vi "Pockels Cal-Init laser power meas.vi"(8 "error in (no error)":errorcluster) -> (0 "error out":errorcluster, 2 "Auto-cancel":bool, 3 "Laser power measrement task":refnum<k21>)   [LabVIEW 2017]
uses:
  Typedefs/HW config states enum.ctl
  <vilib>/DAQmx/create/channels.llb/DAQmx Create Channel (AI-Voltage-Basic).vi
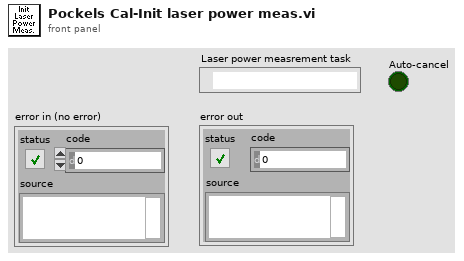
[diagram p1: front panel]
types:
  T1 = typedef "HW config states enum.ctl" = enum16{"Load from file", "Save to file", "Write all", "Read all", "Write XY stage settings", "Write DAQ FPGA settings", "Write Control FPGA settings", "Write Phys Channels", "Clear", "Compare from file"}
  T2 = typedef "Hardware Configuration settings.ctl" = cluster{"Microscope ID":string, "Microscope Type":string, "Revision Number":string, "Advanced Imaging":bool, "Max Allowed Trial Length":dbl, "Initial Scan Resolution":dbl, "Initial Acceptance Angle":dbl, "Dev. PC":bool, "Swap XY on stage":bool, "No of AOD":u8, "MC Supported":bool, "Axial MC":bool, "Computer MAC address":string, "Externalise Triggers":bool, "Trigger HW config":T3, "DAQmx Chan":T4, "XY stage available":bool, "XY Stage":T5, "Z stage available":bool, "Z Stage config cluster":T6, "Encoder available":bool, "Encoder":T7, "VidRec available":bool, "Cam VidRec":T8, "Laser Power Control HW config":T9, "Laser 1 available":bool, "Laser 1 config cluster":T10, "Prechirper 1 available":bool, "Prechirper 1 config cluster":T11, "Control system.FPGA available?":bool, "Control Sys. HW config":T12, "DAQ FPGA HW Config":cluster{"Target":T13, "input card type":T14}}
  T3 = typedef "Triggers HW config.ctl" = cluster{"Available Device List":i32, "Device Address":string}
  T4 = typedef "DAQmx physical channels cluster.ctl" = cluster{"Pockels AO":tag, "Hard shutter AO":tag, "PMT AOs":tag, "Galvo AOs":tag, "Power meter AI":tag}
  T5 = typedef "XY Stage config cluster.ctl" = cluster{"COM port":refnum<visa-resource-name>, "XY stage available":bool, "Baudrate":i32, "Type":string}
  T6 = typedef "Z Stage config cluster.ctl" = cluster{"COM port":refnum<visa-resource-name>, "Z stage available":bool, "Baudrate":i32, "Type":string}
  T7 = typedef "Encoder config cluster.ctl" = cluster{"IP address":string, "Port":u16, "Encoder available":bool, "Wheel radius (cm)":dbl, "Encoder Trigger":tag}
  T8 = typedef "Cam VidRec HW config setup cluster.ctl" = cluster{"DO flag-Video record":tag, "DO flag-Trial start":tag, "VidRec available":bool}
  T9 = typedef "Laser Power Control HW config.ctl" = cluster{"Laser Power Control":string, "Laser Power Modulation Control":string}
  T10 = typedef "Laser 1 config cluster.ctl" = cluster{"COM port":refnum<visa-resource-name>, "Laser 1 available":bool, "Baud Rate":i32, "Type":string}
  T11 = typedef "PreChirper 1 config cluster.ctl" = cluster{"Type":string, "Baud Rate":i32, "Prechirper 1 available":bool, "COM port":refnum<visa-resource-name>}
  T12 = typedef "Control Sys HW config cluster.ctl" = cluster{"Control system.FPGA available?":bool, "Control system.FPGA Type":string, "Control system.Network adapter name":string, "Control system.MAC address":string, "Control system.Ethernet Port":u32}
  T13 = typedef "nirio_resource_hc.ctl" = tag
  T14 = typedef "FPGA input type AC-DC.ctl" = enum16{"AC Card", "DC Card"}
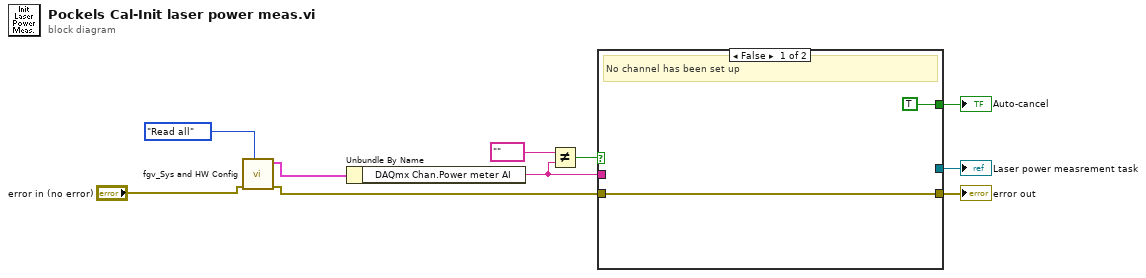
[diagram p0: block diagram]
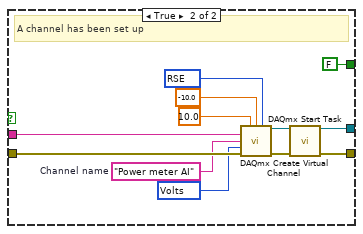
[diagram p2: hidden frame]
diagram:
  n1 = call "fgv_Sys and HW Config.vi"("Function"=HW_config_states_enum."Read all", "error in (no error)"="error in (no error)") -> ("error out"=w3:errorcluster, "Hardware Configuration OUT"=w1:T2)  [unwired: 7 in, 1 out]
  n2 = Unbundle By Name(w1) -> ("DAQmx Chan.Power meter AI"=w8:tag)
  n3 = Not Equal?(x=tag "" ("DAQmx Chan.Power meter AI"), y=w8) -> (x != y?=w6:bool)
  n4 = case shown="False" w6 {
    tunnel: [_ w24] -> w10
    tunnel: [w12 w23] -> w9
    tunnel: w3 -> [w12 w21]
    tunnel: w8 -> [_ w14]
    tunnel: [TRUE FALSE] -> w5
    frame False {
      # "No channel has been set up"
    }
    frame True {
      w19 = "Power meter AI"  # Channel name
      w18 = 10348 items=["Volts"=10348, "From TEDS"=12516, "From Custom Scale"=10065] ("units")
      w15 = 10083 items=["default"=-1, "RSE"=10083, "NRSE"=10078, "Differential"=10106, "Pseudodifferential"=12529] ("input terminal configuration")
      # "A channel has been set up"
      n5 = call-poly <vilib>:"DAQmx Create Virtual Channel.vi"("maximum value"=10.0, "minimum value"=-10.0, "input terminal configuration"=w15, "physical channels"=w14, "name to assign"=w19, "units"=w18, "error in"=w21) -> ("task out"=w20:refnum<k21>, "error out"=w22:errorcluster)  [unwired: 7 in]
      n6 = call <vilib>:"DAQmx Start Task.vi"("task/channels in"=w20, "error in"=w22) -> ("task out"=w24:refnum<k21>, "error out"=w23:errorcluster)  [unwired: 12 in]
    }
  }
  "Laser power measrement task" <- w10
  "error out" <- w9
  "Auto-cancel" <- w5
